vi "tcp_client_Rx_y_Tx_1.vi"() -> ()   [LabVIEW 2020]
panel:
  in  "OK Button 2":bool
  out "Thermometer":dbl(slide) scale=0.0..30.0
  out "match + rest of string":string
  out "substring before match":string
  in  "OK Button":bool
  in  "COMANDO":string
  in  "ENVIAR":bool
  in  "OFF":bool
  in  "ON":bool
  out "Waveform Chart":dbl(graph)
  out "Gauge":dbl(knob) scale=0.0..250.0
  in  "stop":bool
  out "data out":string
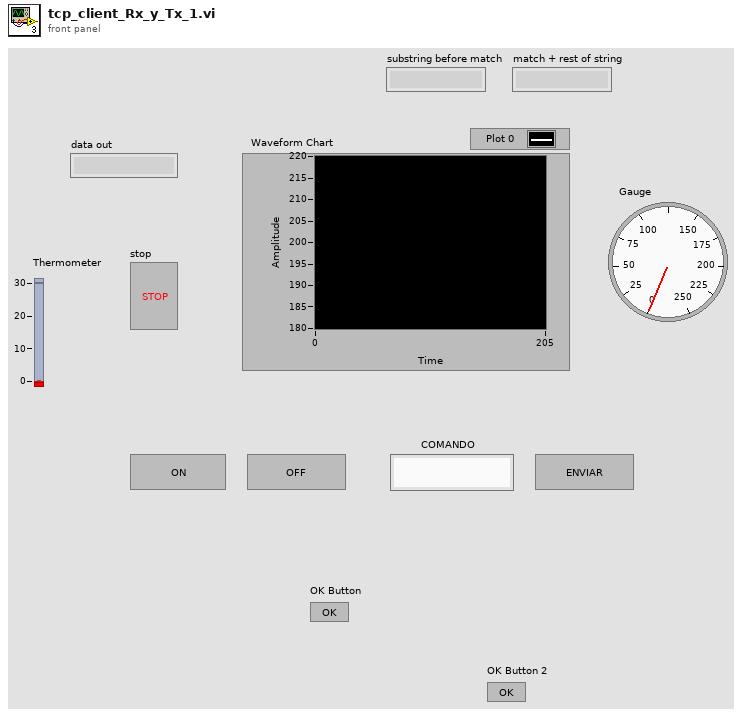
[diagram p1: front panel]
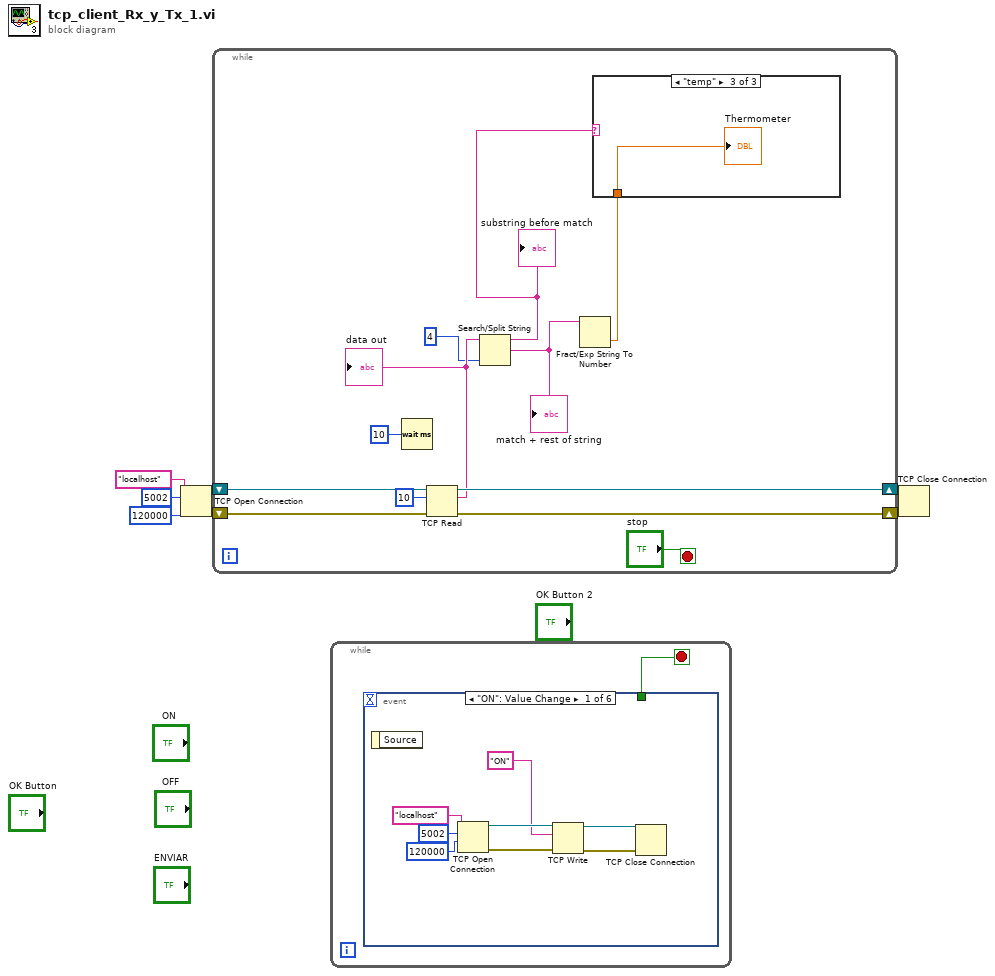
[diagram p0: block diagram]
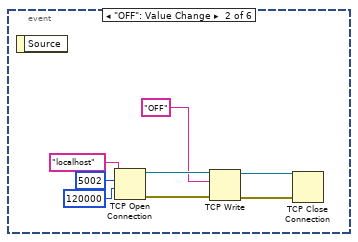
[diagram p2: hidden frame]
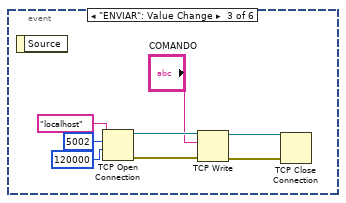
[diagram p3: hidden frame]
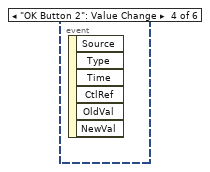
[diagram p4: hidden frame]
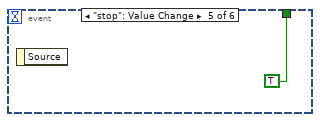
[diagram p5: hidden frame]
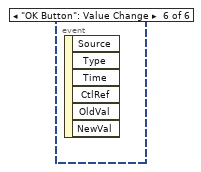
[diagram p6: hidden frame]
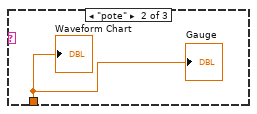
[diagram p8: hidden frame]
diagram:
  n1 = TCP Open Connection(address="localhost", remote port or service name=u16 5002, timeout ms (60000)=120000) -> (connection ID=w2:refnum<k5>, error out=w1:errorcluster)  [unwired: 2 in]
  n2 = while {
    shift-right: [w18] -> w7
    shift-left: w2 -> [w19]
    shift-right: [w16] -> w6
    shift-left: w1 -> [w17]
    stop <- "stop" stop-if-true
    n3 = Wait (ms)(milliseconds to wait=u32 10) -> ()  [unwired: 1 out]
    n4 = TCP Read(connection ID=w19, bytes to read=10, error in (no error)=w17) -> (connection ID out=w18:refnum<k5>, data out=w12:string, error out=w16:errorcluster)  [unwired: 2 in]
    "data out" <- w12
    n5 = Search/Split String(string=w12, offset (0)=4) -> (substring before match=w9:string, match + rest of string=w10:string)  [unwired: 1 in, 1 out]
    "substring before match" <- w9
    "match + rest of string" <- w10
    n6 = Fract/Exp String To Number(string=w10) -> (number=w8:dbl)  [unwired: 3 in, 1 out]
    n7 = case shown="\"temp\"" w9 {
      tunnel: w8 -> [_ w20 w21]
      frame " ", Default {
      }
      frame "pote" {
        "Waveform Chart" <- w20
        "Gauge" <- w20
      }
      frame "temp" {
        "Thermometer" <- w21
      }
    }
  }
  n8 = while {
    stop <- w22 stop-if-true
    n9 = event shown="[0] \"ON\": Value Change" {
      selector: _ -> [_ _ _ _ _ _]
      dyn-events: _ -> [_ _ _ _ _ _]
      timeout: _ -> [_ _ _ _ _ _]
      tunnel: [_ _ _ _ TRUE _] -> w22
      event "ON": Value Change {
        n10 = event-data() -> ()  [unwired: 1 in, 1 out]
        n11 = TCP Open Connection(address="localhost", remote port or service name=u16 5002, timeout ms (60000)=120000) -> (connection ID=w30:refnum<k5>, error out=w29:errorcluster)  [unwired: 2 in]
        n12 = TCP Write(connection ID=w30, data in="ON", error in (no error)=w29) -> (connection ID out=w28:refnum<k5>, error out=w27:errorcluster)  [unwired: 1 in, 1 out]
        n13 = TCP Close Connection(connection ID=w28, error in (no error)=w27) -> ()  [unwired: 1 in, 2 out]
      }
      event "OFF": Value Change {
        n14 = event-data() -> ()  [unwired: 1 in, 1 out]
        n15 = TCP Open Connection(address="localhost", remote port or service name=u16 5002, timeout ms (60000)=120000) -> (connection ID=w38:refnum<k5>, error out=w37:errorcluster)  [unwired: 2 in]
        n16 = TCP Write(connection ID=w38, data in="OFF", error in (no error)=w37) -> (connection ID out=w36:refnum<k5>, error out=w35:errorcluster)  [unwired: 1 in, 1 out]
        n17 = TCP Close Connection(connection ID=w36, error in (no error)=w35) -> ()  [unwired: 1 in, 2 out]
      }
      event "ENVIAR": Value Change {
        n18 = event-data() -> ()  [unwired: 1 in, 1 out]
        n19 = TCP Open Connection(address="localhost", remote port or service name=u16 5002, timeout ms (60000)=120000) -> (connection ID=w43:refnum<k5>, error out=w44:errorcluster)  [unwired: 2 in]
        n20 = TCP Write(connection ID=w43, data in="COMANDO", error in (no error)=w44) -> (connection ID out=w45:refnum<k5>, error out=w46:errorcluster)  [unwired: 1 in, 1 out]
        n21 = TCP Close Connection(connection ID=w45, error in (no error)=w46) -> ()  [unwired: 1 in, 2 out]
      }
      event "OK Button 2": Value Change {
        n22 = event-data() -> ()  [unwired: 1 in, 6 out]
      }
      event "stop": Value Change {
        n23 = event-data() -> ()  [unwired: 1 in, 1 out]
      }
      event "OK Button": Value Change {
        n24 = event-data() -> ()  [unwired: 1 in, 6 out]
      }
    }
  }
  n25 = TCP Close Connection(connection ID=w7, error in (no error)=w6) -> ()  [unwired: 1 in, 2 out]
